vi "Get Or Create Typedef.vi"(8 "error in (no error)":errorcluster, 9 "Create cluster inside Typedef?":bool, 10 "Name":string, 11 "Library in":refnum<vi>) -> (0 "error out":errorcluster, 1 "Cluster ref out":refnum<vi>, 2 "VI ref out":refnum<vi>, 3 "Library out":refnum<vi>, 5 "Path":path)   [LabVIEW 2019, in "gRPC Template Creation Utility.lvlib"]
uses:
  gRPC Template Creation Utility.lvlib
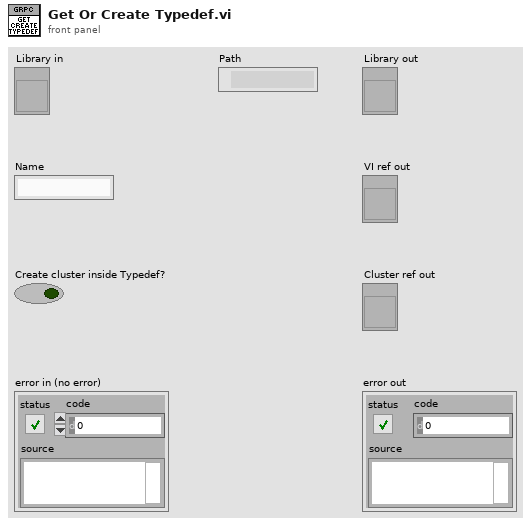
[diagram p1: front panel]
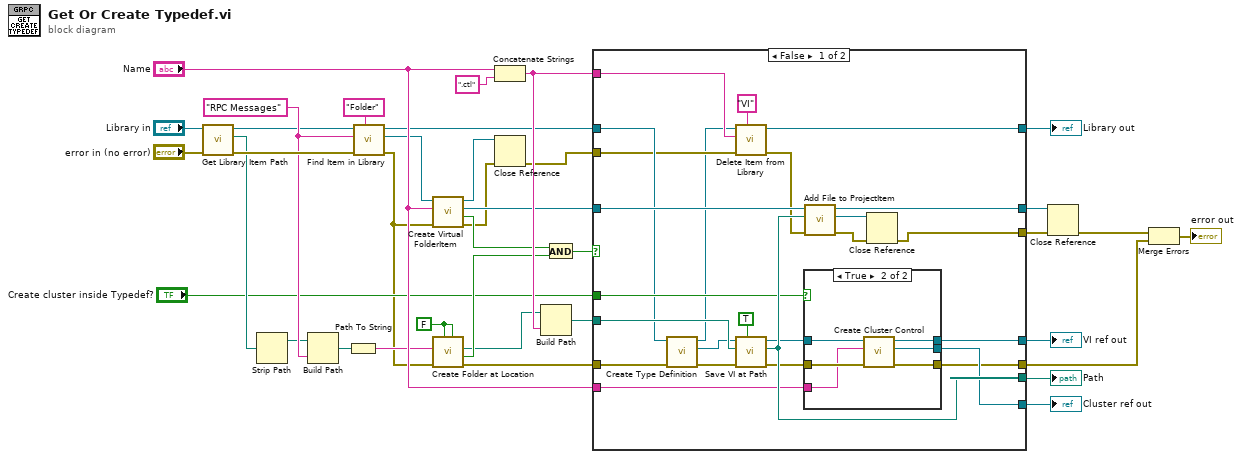
[diagram p0: block diagram]
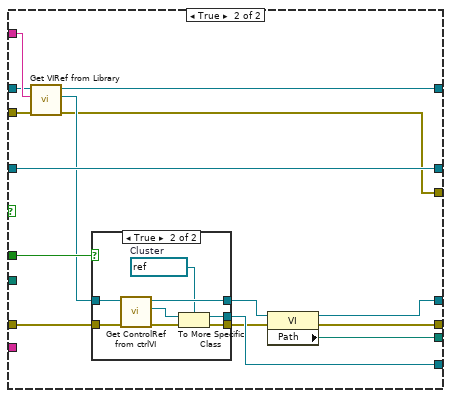
[diagram p3: hidden frame]
diagram:
  w22 = "RPC Messages" ("Item Name")
  w6 = FALSE ("Use Relative")
  n1 = call "Get Library Item Path.vi"("error in (no error)"="error in (no error)", "Library"="Library in") -> ("error out"=w23:errorcluster, "Path"=w16:path, "Library"=w21:refnum<vi>)  [unwired: 7 in]
  n2 = Strip Path(path=w16) -> (stripped path=w15:path)  [unwired: 1 out]
  n3 = Build Path(base path=w15, name or relative path=w22) -> (appended path=w36:path)
  n4 = Path To String(path=w36) -> (string=w13:string)
  n5 = call "Find Item in Library.vi"("Item Type"="Folder", "error in (no error)"=w23, "Item Name"=w22, "Library item in"=w21) -> ("error out"=w1:errorcluster, "Project Item (Library Item)"=w20:refnum<vi>, "Library item out"=w27:refnum<vi>)  [unwired: 4 in, 1 out]
  n6 = call "Create Virtual FolderItem.vi"("error in (no error)"=w1, "Folder Name"="Name", "ProjectItem in"=w20) -> ("error out"=w4:errorcluster, "Already exists?"=w30:bool, "FolderItem reference out"=w26:refnum<vi>, "ProjectItem out"=w3:refnum<vi>)  [unwired: 5 in]
  n7 = call "Create Folder at Location.vi"("Override existing (F)"=w6, "Use Relative (F)"=w6, "Error In"=w1, "Path"=w13) -> ("Error Out"=w14:errorcluster, "Already Exists ?"=w31:bool, "Full path out"=w12:path)  [unwired: 5 in]
  n8 = Concatenate Strings("Name", ".ctl" ("string")) -> (w34:string)
  n9 = Close Reference(reference=w3, error in (no error)=w4) -> (error out=w2:errorcluster)
  n10 = Build Path(base path=w12, name or relative path=w34) -> (appended path=w25:path)
  n11 = And(x=w30, y=w31) -> (x .and. y?=w32:bool)
  n12 = case shown="False" w32 {
    tunnel: w14 -> [w62 w73]
    tunnel: [w45 w83] -> w18
    tunnel: [w61 w76] -> w37
    tunnel: [w60 w71] -> w9
    tunnel: w25 -> [w59 _]
    tunnel: w26 -> [w57 w81]
    tunnel: w27 -> [w40 w80]
    tunnel: [w42 w85] -> w28
    tunnel: [w55 w81] -> w11
    tunnel: w34 -> [w50 w82]
    tunnel: [w56 w84] -> w29
    tunnel: w2 -> [w39 w74]
    tunnel: [w54 w72] -> w10
    tunnel: "Name" -> [w47 _]
    tunnel: "Create cluster inside Typedef?" -> [w46 w79]
    frame False {
      n13 = call "Create Type Definition.vi"("error in (no error)"=w62, "library in"=w40) -> ("error out"=w58:errorcluster, "TypeDef VI out"=w41:refnum<vi>, "library out"=w38:refnum<vi>)  [unwired: 7 in]
      n14 = call "Delete Item from Library.vi"("Item Type"="VI", "error in (no error)"=w39, "Item name"=w50, "Library"=w38) -> ("error out"=w49:errorcluster, "Library"=w42:refnum<vi>)  [unwired: 5 in, 1 out]
      n15 = call "Save VI at Path.vi"("Override Existing? (T)"=TRUE, "error in (no error)"=w58, "Path"=w59, "VI in"=w41) -> ("error out"=w53:errorcluster, "Path to saved File"=w56:path, "VI out"=w52:refnum<vi>)  [unwired: 5 in]
      n16 = case shown="True" w46 {
        tunnel: [_ w70] -> w61
        tunnel: [w64 w69] -> w60
        tunnel: w53 -> [w64 w68]
        tunnel: w52 -> [w63 w67]
        tunnel: w47 -> [_ w66]
        tunnel: [w63 w65] -> w45
        frame False {
        }
        frame True {
          n17 = call "Create Cluster Control.vi"("error in (no error)"=w68, "Cluster Label"=w66, "Owning vi in"=w67) -> ("error out"=w69:errorcluster, "Cluster ref out"=w70:refnum<vi>, "Owning vi out"=w65:refnum<vi>)  [unwired: 6 in]
        }
      }
      n18 = call "Add File to ProjectItem.vi"("error in (no error)"=w49, "File Path"=w56, "ProjectItem in"=w57) -> ("error out"=w43:errorcluster, "Added File ref"=w44:refnum<vi>, "ProjectItem out"=w55:refnum<vi>)  [unwired: 6 in]
      n19 = Close Reference(reference=w44, error in (no error)=w43) -> (error out=w54:errorcluster)
    }
    frame True {
      n20 = call "Get VIRef from Library.vi"("error in (no error)"=w74, "item name"=w82, "library in"=w80) -> ("error out"=w72:errorcluster, "vi"=w78:refnum<vi>, "library out"=w85:refnum<vi>)  [unwired: 5 in, 1 out]
      n21 = case shown="True" w79 {
        tunnel: w73 -> [w86 w95]
        tunnel: w78 -> [w87 w94]
        tunnel: [w87 w92] -> w77
        tunnel: [_ w89] -> w76
        tunnel: [w86 w88] -> w75
        frame False {
        }
        frame True {
          w91 = refnum<vi> refnum  # Cluster
          n22 = call "Get ControlRef from ctrlVI.vi"("error in (no error)"=w95, "VI ref in"=w94) -> ("error out"=w93:errorcluster, "Control ref out"=w90:refnum<vi>, "VI ref out"=w92:refnum<vi>)  [unwired: 7 in]
          n23 = To More Specific Class(target class=w91, reference=w90, error in=w93) -> (specific class reference=w89:refnum<vi>, error out=w88:errorcluster)
        }
      }
      n24 = property class="VI"(reference=w77, error in=w75) -> (reference out=w83:refnum<vi>, error out=w71:errorcluster, "Path"=w84:path)
    }
  }
  "Cluster ref out" <- w37
  "Path" <- w29
  "Library out" <- w28
  "VI ref out" <- w18
  n25 = Close Reference(reference=w11, error in (no error)=w10) -> (error out=w5:errorcluster)
  n26 = Merge Errors(w5, w9) -> (→"error out":errorcluster)
